vi "9470 Example FPGA Code.vi"() -> ()   [LabVIEW 2023]
uses:
  <vilib>/LabVIEW Targets/FPGA/cRIO/shared/nicrio_ModuleControls/nicrio_cRIO-9470_DataRatesRing.ctl
  <vilib>/LabVIEW Targets/FPGA/cRIO/shared/nicrio_ModuleControls/nicrio_cRIO-9470_OutputModeRing.ctl
  <vilib>/rvi/Emulation/niFpgaGetClockAttributes.vi
  <vilib>/rvi/Emulation/niFpgaSctlEmulationGetInTimedLoop.vi
  <vilib>/rvi/Emulation/niFpgaEmulationReportErrorSimple.vi
  <vilib>/rvi/Emulation/niFpgaCriticalErrorInLSC.vi
  <vilib>/rvi/eio/common/nirviEmuTemplatePropertySet_noerrors.vi
  <vilib>/rvi/eio/common/nirviEmuTemplateMethod_errors.vi
  <vilib>/eio/utilities/niEioResolveVilibRelativePath.vi
  <vilib>/rvi/interface/RandomDataEmulation/niFpgaRandomDataHandleErrors.vi
  <vilib>/rvi/Emulation/niFpgaProcessEmulError.vi
  <vilib>/eio/EIOPropertyNode/EIOPropertyNode.xnode
  <vilib>/eio/EIOMethodNode/EIOMethodNode.xnode
  <vilib>/eio/EIONode/EIONode.xnode
  <vilib>/rvi/DataTransferAndStorage/Container/XNode/niFpgaContainer.xnode
  <vilib>/rvi/interface/RandomDataEmulation/nirviRandomDataFpgaReadWriteTemplate.vi
  <vilib>/rvi/eio/common/nirviEmuTemplatePropertyGet_errors.vi
  <vilib>/rvi/eio/common/nirviEmuTemplatePropertyGet_noerrors.vi
  <vilib>/rvi/eio/common/nirviEmuTemplatePropertySet_errors.vi
panel:
  out "CH0 Pwr Fault":bool
  out "Module Overtemp":bool
  out "CH0 Overcurrent":bool
  out "CH1 Overcurrent":bool
  out "CH1 Pwr Fault":bool
  in  "stop":bool
  in  "Duty Cycle %":fxp<+,17,7>[](array[numeric])=[0.0, 0.0, 0.0, 0.0, 0.0, 0.0, 0.0, 0.0]
  out "error out":errorcluster
  out "FIFO Timeout":bool
  in  "CH1 Enable on Fault":bool
  in  "CH0 Enable on Fault":bool
  out "Voltage (V)":fxp<+,12,6>[](array[numeric])
  out "Module Temperature":fxp<+/-,12,9>
  in  "PWM Divisor":u16
  in  "Dither Amplitude":fxp<+,17,7>
  in  "Dither Divisor":u16
  in  "Data Rate":T1 items=["3.200 kS/s (NI 9470)", "3.125 kS/s (NI 9470)", "2.560 kS/s (NI 9470)", "2.000 kS/s (NI 9470)"]
  in  "Ready?":bool
  in  "Application Mode":T2(ring)
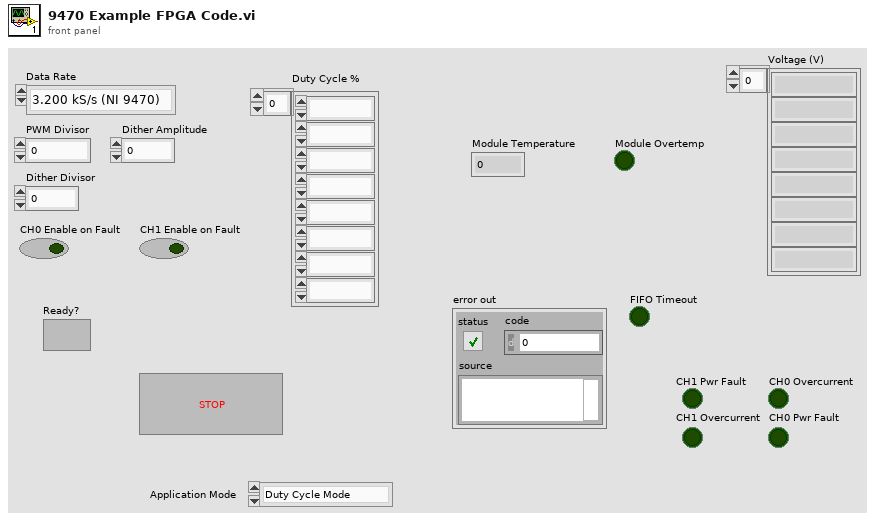
[diagram p1: front panel]
types:
  T1 = typedef "nicrio_cRIO-9470_DataRatesRing.ctl" = u8
  T2 = enum16{"Duty Cycle Mode", "Average Current Mode"}
  T3 = typedef "nicrio_cRIO-9470_OutputModeRing.ctl" = u8
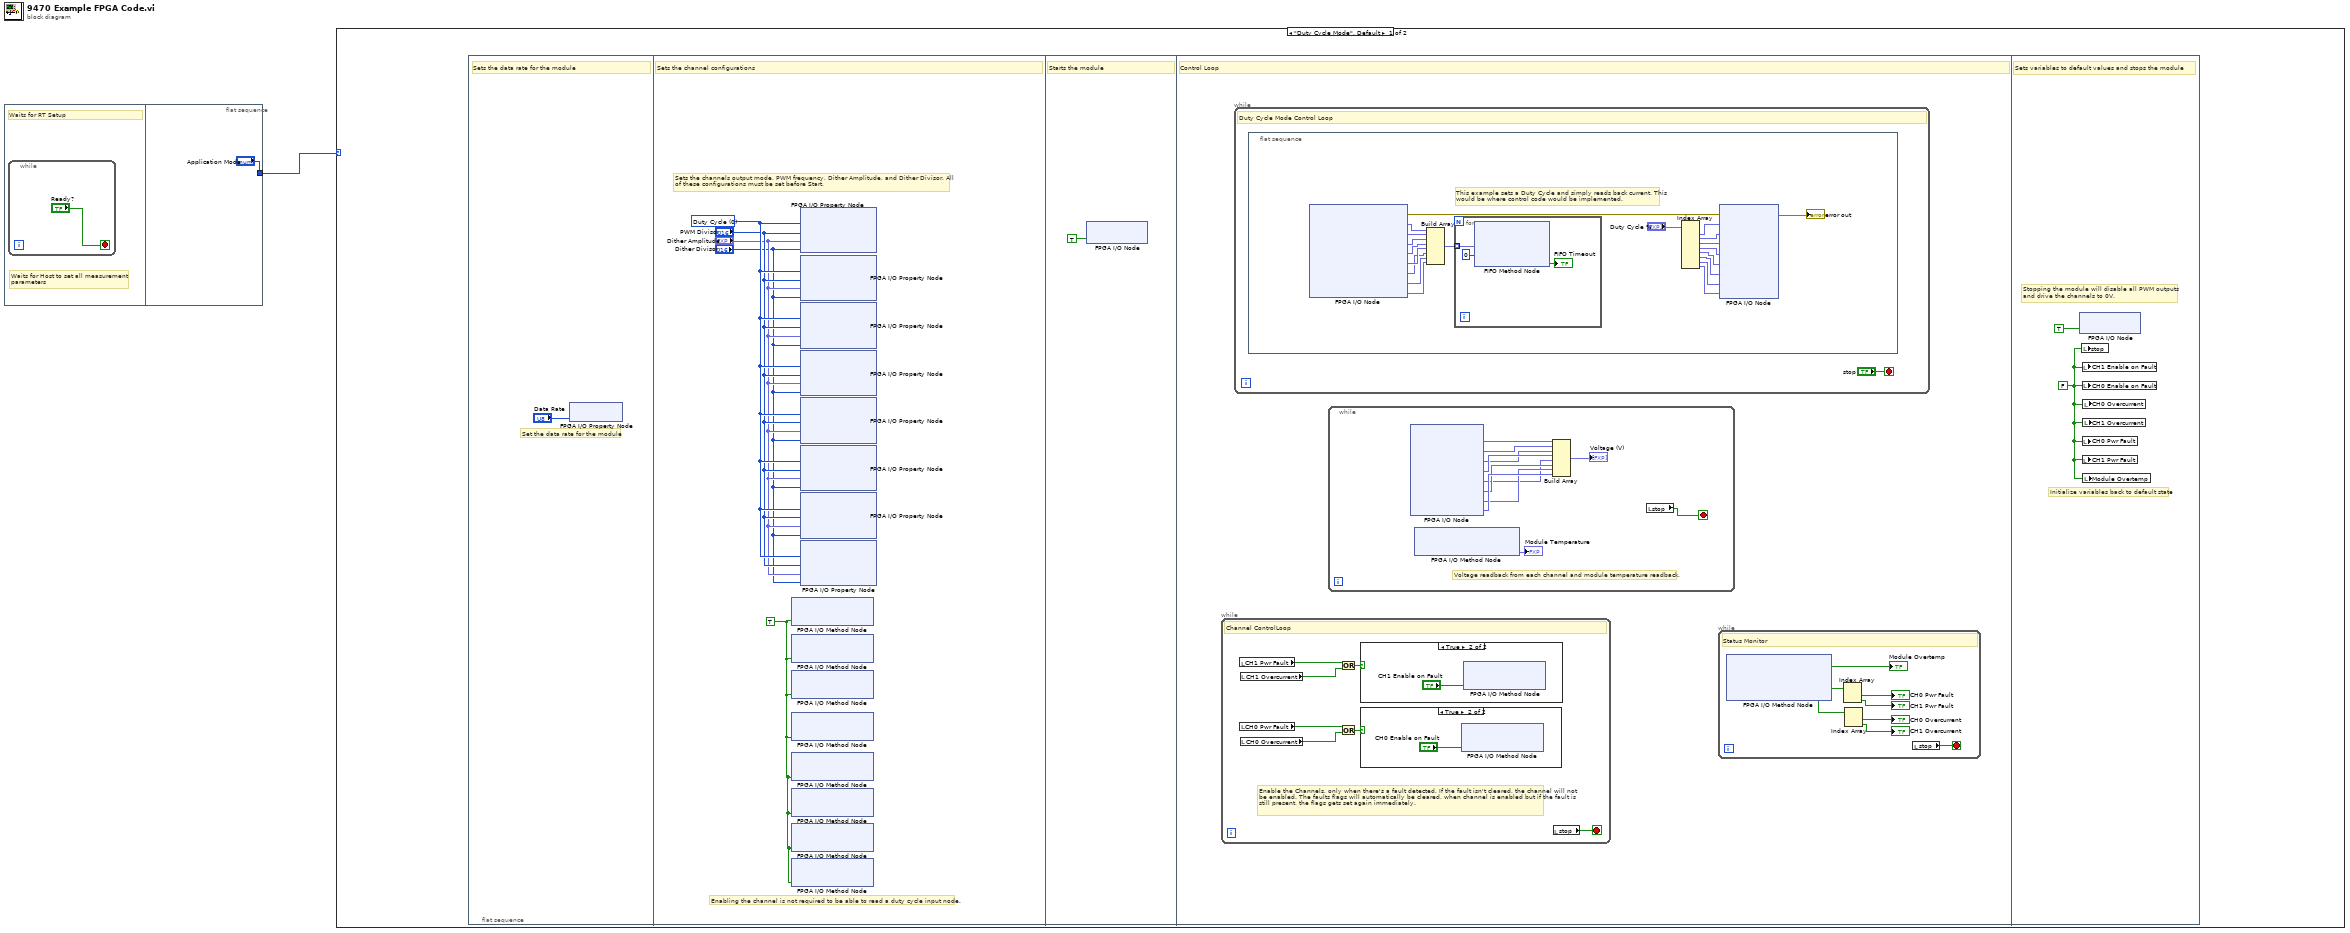
[diagram p0: block diagram]
diagram:
  n1 = flat-sequence {
    tunnel: ["Application Mode"] -> w1
    frame #0 {
      # "Waits for Host to set all measurement \nparameters"
      # "Waits for RT Setup"
      n2 = while {
        stop <- "Ready?" stop-if-true
      }
    }
    frame #1 {
    }
  }
  n3 = case shown="\"Duty Cycle Mode\", Default" w1 {
    frame "Duty Cycle Mode", Default {
      n4 = flat-sequence {
        frame #0 {
          # "Set the data rate for the module"
          # "Sets the data rate for the module"
          n5 = xnode "FPGA I/O Property Node"("Data Rate"="Data Rate") -> ()  [unwired: 1 in, 1 out]
        }
        frame #1 {
          w9 = T3 0 items=["Duty Cycle", "Average Current"] ("Output Mode")
          w7 = TRUE ("Enable")
          # "Enabling the channel is not required to be able to read a duty cycle input node."
          # "Sets the channels output mode, PWM frequency, Dither Amplitude, and Dither Divisor. All\nof these configurations must be set before Start."
          # "Sets the channel configurations"
          n6 = xnode "FPGA I/O Method Node"("Enable"=w7) -> ()  [unwired: 1 in, 1 out]
          n7 = xnode "FPGA I/O Method Node"("Enable"=w7) -> ()  [unwired: 1 in, 1 out]
          n8 = xnode "FPGA I/O Method Node"("Enable"=w7) -> ()  [unwired: 1 in, 1 out]
          n9 = xnode "FPGA I/O Method Node"("Enable"=w7) -> ()  [unwired: 1 in, 1 out]
          n10 = xnode "FPGA I/O Method Node"("Enable"=w7) -> ()  [unwired: 1 in, 1 out]
          n11 = xnode "FPGA I/O Method Node"("Enable"=w7) -> ()  [unwired: 1 in, 1 out]
          n12 = xnode "FPGA I/O Method Node"("Enable"=w7) -> ()  [unwired: 1 in, 1 out]
          n13 = xnode "FPGA I/O Method Node"("Enable"=w7) -> ()  [unwired: 1 in, 1 out]
          n14 = xnode "FPGA I/O Property Node"("Output Mode"=w9, "PWM Divisor"="PWM Divisor", "Dither Amplitude"="Dither Amplitude", "Dither Divisor"="Dither Divisor") -> ()  [unwired: 1 in, 1 out]
          n15 = xnode "FPGA I/O Property Node"("Output Mode"=w9, "PWM Divisor"="PWM Divisor", "Dither Amplitude"="Dither Amplitude", "Dither Divisor"="Dither Divisor") -> ()  [unwired: 1 in, 1 out]
          n16 = xnode "FPGA I/O Property Node"("Output Mode"=w9, "PWM Divisor"="PWM Divisor", "Dither Amplitude"="Dither Amplitude", "Dither Divisor"="Dither Divisor") -> ()  [unwired: 1 in, 1 out]
          n17 = xnode "FPGA I/O Property Node"("Output Mode"=w9, "PWM Divisor"="PWM Divisor", "Dither Amplitude"="Dither Amplitude", "Dither Divisor"="Dither Divisor") -> ()  [unwired: 1 in, 1 out]
          n18 = xnode "FPGA I/O Property Node"("Output Mode"=w9, "PWM Divisor"="PWM Divisor", "Dither Amplitude"="Dither Amplitude", "Dither Divisor"="Dither Divisor") -> ()  [unwired: 1 in, 1 out]
          n19 = xnode "FPGA I/O Property Node"("Output Mode"=w9, "PWM Divisor"="PWM Divisor", "Dither Amplitude"="Dither Amplitude", "Dither Divisor"="Dither Divisor") -> ()  [unwired: 1 in, 1 out]
          n20 = xnode "FPGA I/O Property Node"("Output Mode"=w9, "PWM Divisor"="PWM Divisor", "Dither Amplitude"="Dither Amplitude", "Dither Divisor"="Dither Divisor") -> ()  [unwired: 1 in, 1 out]
          n21 = xnode "FPGA I/O Property Node"("Output Mode"=w9, "PWM Divisor"="PWM Divisor", "Dither Amplitude"="Dither Amplitude", "Dither Divisor"="Dither Divisor") -> ()  [unwired: 1 in, 1 out]
        }
        frame #2 {
          # "Starts the module"
          n22 = xnode "FPGA I/O Node"("Mod3/Start"=TRUE ("Mod1/Start")) -> ()  [unwired: 1 in, 1 out]
        }
        frame #3 {
          # "Control Loop"
          n23 = while {
            stop <- w28 stop-if-true
            # "Enable the Channels, only when there's a fault detected. If the fault isn't cleared, the channel will not be enabled. The faults flags will automatically be cleared, when channel is enabled but if the fault is still present, the flags gets set again immediately."
            # "Channel ControlLoop"
            n24 = local read "CH1 Pwr Fault"() -> (w26:bool)
            n25 = local read "CH0 Pwr Fault"() -> (w23:bool)
            n26 = local read "CH1 Overcurrent"() -> (w25:bool)
            n27 = local read "CH0 Overcurrent"() -> (w24:bool)
            n28 = Or(x=w23, y=w24) -> (x .or. y?=w22:bool)
            n29 = Or(x=w26, y=w25) -> (x .or. y?=w27:bool)
            n30 = case shown="True" w27 {
              frame False {
              }
              frame True {
                n31 = xnode "FPGA I/O Method Node"("Enable"="CH1 Enable on Fault") -> ()  [unwired: 1 in, 1 out]
              }
            }
            n32 = case shown="True" w22 {
              frame False {
              }
              frame True {
                n33 = xnode "FPGA I/O Method Node"("Enable"="CH0 Enable on Fault") -> ()  [unwired: 1 in, 1 out]
              }
            }
            n34 = local read "stop"() -> (w28:bool)
          }
          n35 = while {
            stop <- "stop" stop-if-true
            # "Duty Cycle Mode Control Loop"
            n36 = flat-sequence {
              frame #0 {
                # "This example sets a Duty Cycle and simply reads back current. This\nwould be where control code would be implemented."
                n37 = xnode "FPGA I/O Node"() -> ("error out"=w49:errorcluster, "Mod3/AverageCurrent0"=w51:fxp<+/-,16,3>, "Mod3/AverageCurrent1"=w46:fxp<+/-,16,3>, "Mod3/AverageCurrent2"=w45:fxp<+/-,16,3>, "Mod3/AverageCurrent3"=w44:fxp<+/-,16,3>, "Mod3/AverageCurrent4"=w43:fxp<+/-,16,3>, "Mod3/AverageCurrent5"=w42:fxp<+/-,16,3>, "Mod3/AverageCurrent6"=w41:fxp<+/-,16,3>, "Mod3/AverageCurrent7"=w40:fxp<+/-,16,3>)  [unwired: 9 in, 8 out]
                n38 = Build Array(w51, w46, w45, w44, w43, w42, w41, w40) -> (w47:fxp<+/-,16,3>[])
                n39 = for {
                  tunnel: w47 -> [w54] mode=indexing
                  n40 = xnode ("FIFO Method Node")("Element"=w54, "Timeout"=0) -> ("Timed Out?"=→"FIFO Timeout":bool)  [unwired: 1 in, 1 out]
                }
                n41 = Index Array(array="Duty Cycle %") -> (element #1=w39:fxp<+,17,7>, element #2=w38:fxp<+,17,7>, element #3=w37:fxp<+,17,7>, element #4=w36:fxp<+,17,7>, element #5=w35:fxp<+,17,7>, element #6=w34:fxp<+,17,7>, element #7=w33:fxp<+,17,7>, element #8=w32:fxp<+,17,7>)  [unwired: 8 in]
                n42 = xnode "FPGA I/O Node"("error in"=w49, "Mod3/CH0"=w39, "Mod3/CH1"=w38, "Mod3/CH2"=w37, "Mod3/CH3"=w36, "Mod3/CH4"=w35, "Mod3/CH5"=w34, "Mod3/CH6"=w33, "Mod3/CH7"=w32) -> ("error out"=→"error out":errorcluster)  [unwired: 8 in, 8 out]
              }
            }
          }
          n43 = while {
            stop <- w21 stop-if-true
            # "Voltage readback from each channel and module temperature readback."
            n44 = xnode "FPGA I/O Node"() -> ("Mod3/Voltage0"=w11:fxp<+,12,6>, "Mod3/Voltage1"=w12:fxp<+,12,6>, "Mod3/Voltage2"=w13:fxp<+,12,6>, "Mod3/Voltage3"=w14:fxp<+,12,6>, "Mod3/Voltage4"=w15:fxp<+,12,6>, "Mod3/Voltage5"=w16:fxp<+,12,6>, "Mod3/Voltage6"=w17:fxp<+,12,6>, "Mod3/Voltage7"=w18:fxp<+,12,6>)  [unwired: 8 in, 8 out]
            n45 = xnode "FPGA I/O Method Node"() -> ("Module Temperature"=→"Module Temperature":fxp<+/-,12,9>)  [unwired: 1 in, 1 out]
            n46 = Build Array(w11, w12, w13, w14, w15, w16, w17, w18) -> (→"Voltage (V)":fxp<+,12,6>[])
            n47 = local read "stop"() -> (w21:bool)
          }
          n48 = while {
            stop <- w62 stop-if-true
            # "Status Monitor"
            n49 = xnode "FPGA I/O Method Node"() -> ("Module Over Temperature"=→"Module Overtemp":bool, "Power Supply Fault"=w60:bool[], "Channel Overcurrent"=w57:bool[])  [unwired: 1 in, 1 out]
            n50 = Index Array(array=w60) -> (element #1=→"CH0 Pwr Fault":bool, element #2=→"CH1 Pwr Fault":bool)  [unwired: 2 in]
            n51 = Index Array(array=w57) -> (element #1=→"CH0 Overcurrent":bool, element #2=→"CH1 Overcurrent":bool)  [unwired: 2 in]
            n52 = local read "stop"() -> (w62:bool)
          }
        }
        frame #4 {
          w64 = FALSE ("CH1 Timeout")
          # "Stopping the module will disable all PWM outputs\nand drive the channels to 0V."
          # "Initialize variables back to default state"
          # "Sets variables to default values and stops the module"
          n53 = xnode "FPGA I/O Node"("Mod3/Stop"=TRUE ("9470/Start")) -> ()  [unwired: 1 in, 1 out]
          n54 = local write "stop"(w64) -> ()
          n55 = local write "CH1 Enable on Fault"(w64) -> ()
          n56 = local write "CH0 Enable on Fault"(w64) -> ()
          n57 = local write "CH0 Pwr Fault"(w64) -> ()
          n58 = local write "CH1 Pwr Fault"(w64) -> ()
          n59 = local write "CH0 Overcurrent"(w64) -> ()
          n60 = local write "CH1 Overcurrent"(w64) -> ()
          n61 = local write "Module Overtemp"(w64) -> ()
        }
      }
    }
    frame "Average Current Mode" {
    }
  }
